vi "DetalleTanque.vi"() -> ()   [LabVIEW 2018]
panel:
  out "NSV":dbl format="%#_g %%"
  out "GSV":dbl format="%#_g %%"
  out "GOV":dbl format="%#_g %%"
  out "TOV":dbl format="%#_g %%"
  out "Time":string="12:00 p.m."
  out "Date":string="9/24/2020"
  out "Last Event":string="Filling"
  out "Diameter":dbl
  out "Height":dbl
  out "Indicadores Detallados":T1 {"Pressure" format="%#_g psi"; "Fuel Level" format="%#_g L"; "Temperature" format="%#_g °C"; "Percentage" format="%#_g %%"}
  out "Title":string
  in  "stop":bool
  out "Tank":dbl(slide) scale=0.0..100.0 scale format="%#_g%%"
  # "Detailed Metrics"
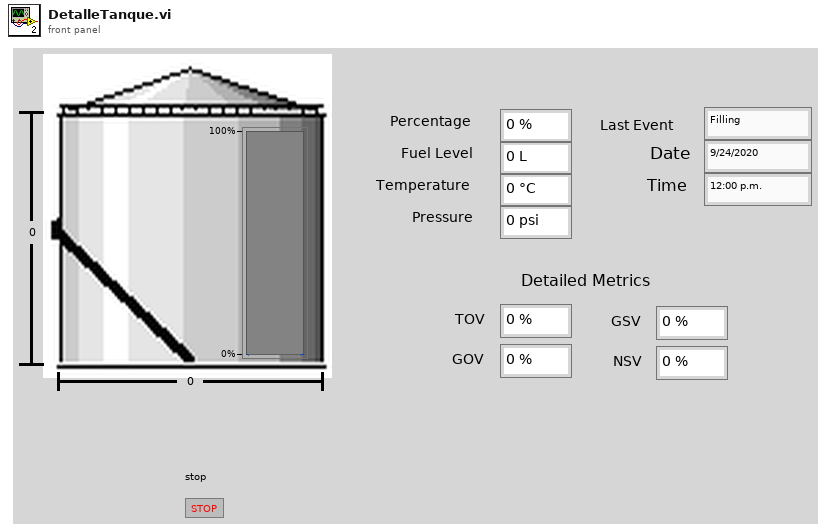
[diagram p1: front panel]
types:
  T1 = cluster{"Pressure":dbl, "Fuel Level":dbl, "Temperature":dbl, "Percentage":dbl}
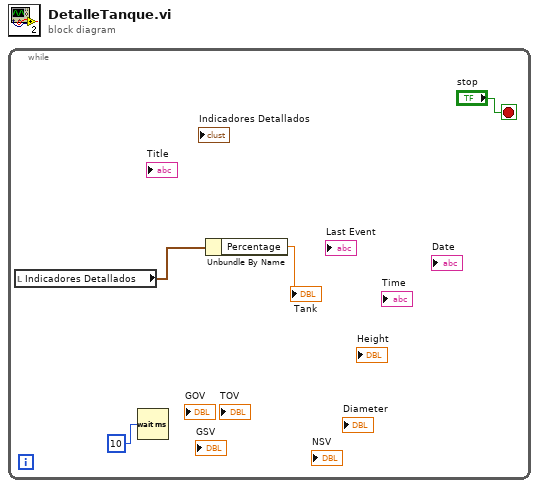
[diagram p0: block diagram]
diagram:
  n1 = while {
    stop <- "stop" stop-if-true
    n2 = local read "Indicadores Detallados"() -> (w2:T1)
    n3 = Wait (ms)(milliseconds to wait=u32 10) -> ()  [unwired: 1 out]
    n4 = Unbundle By Name(w2) -> ("Percentage"=→"Tank":dbl)
  }
